vi "libssh2_channel_read_ex.vi"(8 "error in (no error)":errorcluster, 9 "buflen":u64=1024, 10 "stream_id":i32, 11 "channel":u64) -> (0 "error out":errorcluster, 2 "buf":string, 3 "return value":u64)   [LabVIEW 2013, in "libssh2.lvlib"]
uses:
  libssh2.lvlib
  libssh2.dll
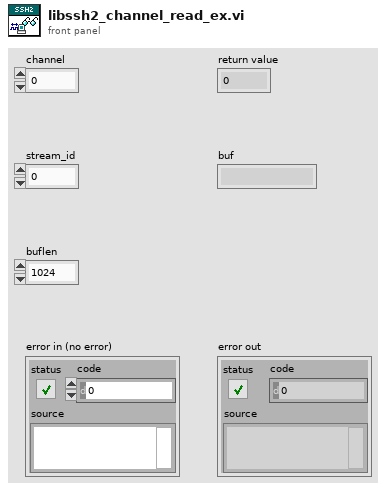
[diagram p1: front panel]
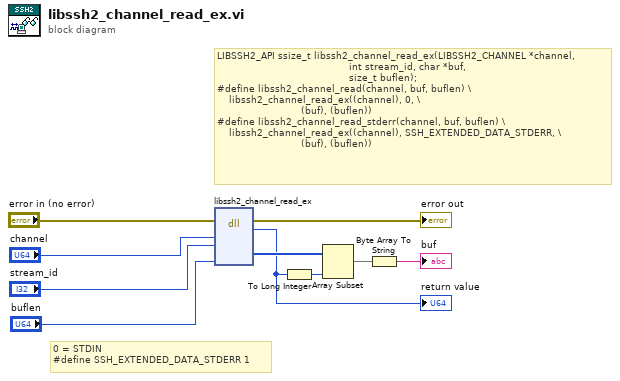
[diagram p0: block diagram]
diagram:
  # "0 = STDIN\n#define SSH_EXTENDED_DATA_STDERR 1"
  # "LIBSSH2_API ssize_t libssh2_channel_read_ex(LIBSSH2_CHANNEL *channel,\n                                            int stream_id, char *buf,\n                                            size_t buflen);\n#define libssh2_channel_read(channel, buf, buflen) \\\n    libssh2_channel_read_ex((channel), 0, \\\n                            (buf), (buflen))\n#define libssh2_channel_read_stderr(channel, buf, buflen) \\\n    libssh2_channel_read_ex((channel), SSH_EXTENDED_DATA_STDERR, \\\n                            (buf), (buflen))"
  n1 = dll-call lib="C:/Users/pasca/source/repos/libssh2-labview/libssh2**.*" fn="libssh2_channel_read_ex"(error in="error in (no error)", "channel"="channel", "stream_id"="stream_id", "buflen"="buflen") -> (error out=→"error out":errorcluster, "return value"=w2:u64, "buf"=w4:u8[])  [unwired: 6 in, 1 out]
  "return value" <- w2
  n2 = To Long Integer(number=w2) -> (32bit integer=w1:i32)
  n3 = Array Subset(array=w4, length=w1) -> (w3:u8[])  [unwired: 1 in]
  n4 = Byte Array To String(unsigned byte array=w3) -> (string=→"buf":string)
